vi "Control Cluster to U16.vi"(11 "Controlword":T1) -> (2 "Control word Data":u8[](array[numeric]), 3 "Controlword U16":u16, 5 "address":u16 format="%04x")   [LabVIEW 2016, in "IgusMotorDrive.lvclass"]
uses:
  IgusMotorDrive.lvclass
  typedefs/Controlword--cluster.ctl
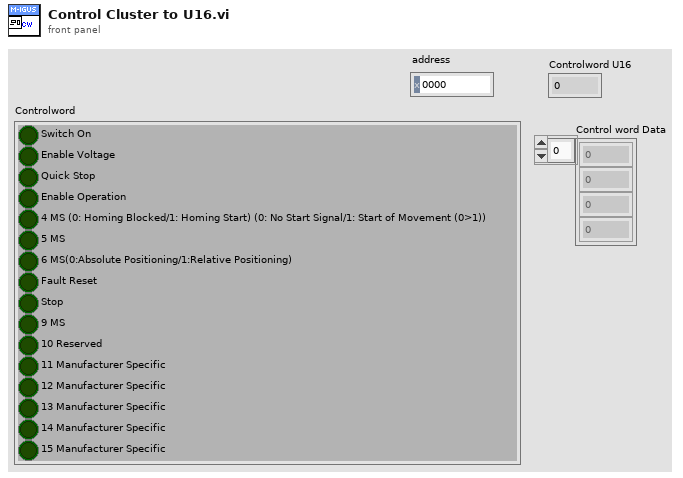
[diagram p1: front panel]
types:
  T1 = typedef "IgusMotorDrive.lvclass/Controlword--cluster.ctl" = cluster{"Switch On":bool, "Enable Voltage":bool, "Quick Stop":bool, "Enable Operation":bool, "4 MS (0: Homing Blocked/1: Homing Start) (0: No Start Signal/1: Start of Movement (0>1))":bool, "5 MS":bool, "6 MS(0:Absolute Positioning/1:Relative Positioning)":bool, "Fault Reset":bool, "Stop":bool, "9 MS":bool, "10 Reserved":bool, "11 Manufacturer Specific":bool, "12 Manufacturer Specific":bool, "13 Manufacturer Specific":bool, "14 Manufacturer Specific":bool, "15 Manufacturer Specific":bool}
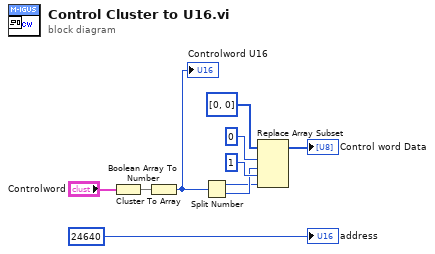
[diagram p0: block diagram]
diagram:
  n1 = Cluster To Array(cluster="Controlword") -> (array=w9:bool[])
  n2 = Boolean Array To Number(Boolean array=w9) -> (number=w2:u16)
  "Controlword U16" <- w2
  n3 = Split Number(x=w2) -> (hi(x)=w4:u8, lo(x)=w5:u8)
  n4 = Replace Array Subset(array=u8[] [0, 0] ("Data [1-4]"), new element #1=w5, index #1=0 ("index"), new element #2=w4, index #2=1 ("index")) -> (→"Control word Data":u8[])
  "address" <- u16 24640 ("address")
